vi "DecodePacket.vi"(0 "object in":refnum<class "Referee.lvclass">, 2 "element":u8[](array[numeric]), 5 "error in (no error)":errorcluster) -> (14 "object out":refnum<class "Referee.lvclass">, 16 "Packet out":T1, 19 "error out":errorcluster)   [LabVIEW 2023, in "Referee.lvclass"]
uses:
  Referee.lvclass
  Packet.ctl
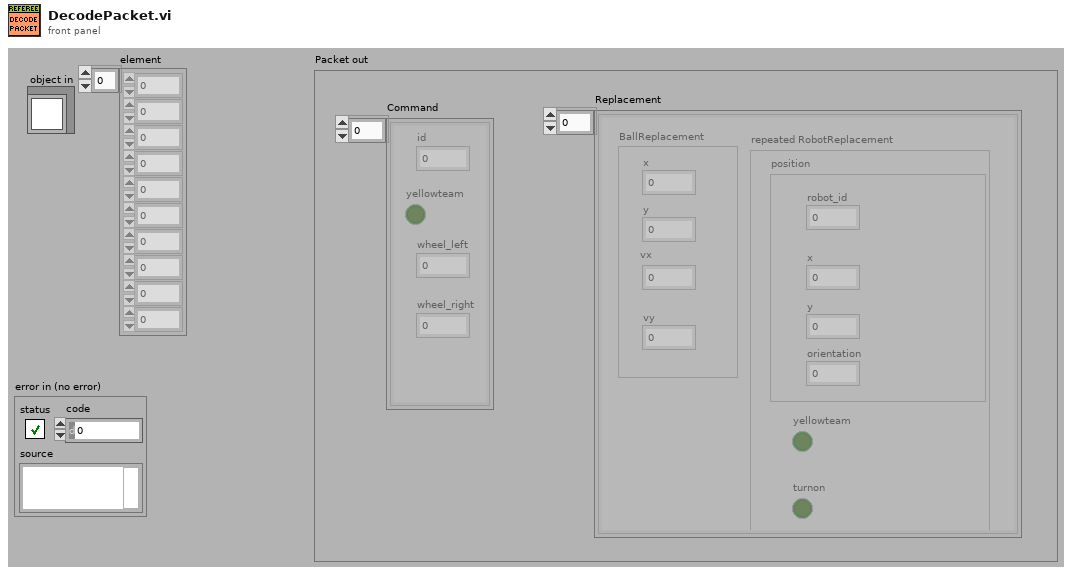
[diagram p1: front panel]
types:
  T1 = typedef "Referee.lvclass/Packet.ctl" = cluster{"Command":cluster{"id":dbl, "yellowteam":bool, "wheel_left":dbl, "wheel_right":dbl}[], "Replacement":cluster{"BallReplacement":cluster{"x":dbl, "y":dbl, "vx":dbl, "vy":dbl}, "repeated RobotReplacement":cluster{"position":cluster{"robot_id":dbl, "x":dbl, "y":dbl, "orientation":dbl}, "yellowteam":bool, "turnon":bool}}[]}
  T2 = cluster{"id":dbl, "yellowteam":bool, "wheel_left":dbl, "wheel_right":dbl}[]
  T3 = cluster{"BallReplacement":cluster{"x":dbl, "y":dbl, "vx":dbl, "vy":dbl}, "repeated RobotReplacement":cluster{"position":cluster{"robot_id":dbl, "x":dbl, "y":dbl, "orientation":dbl}, "yellowteam":bool, "turnon":bool}}[]
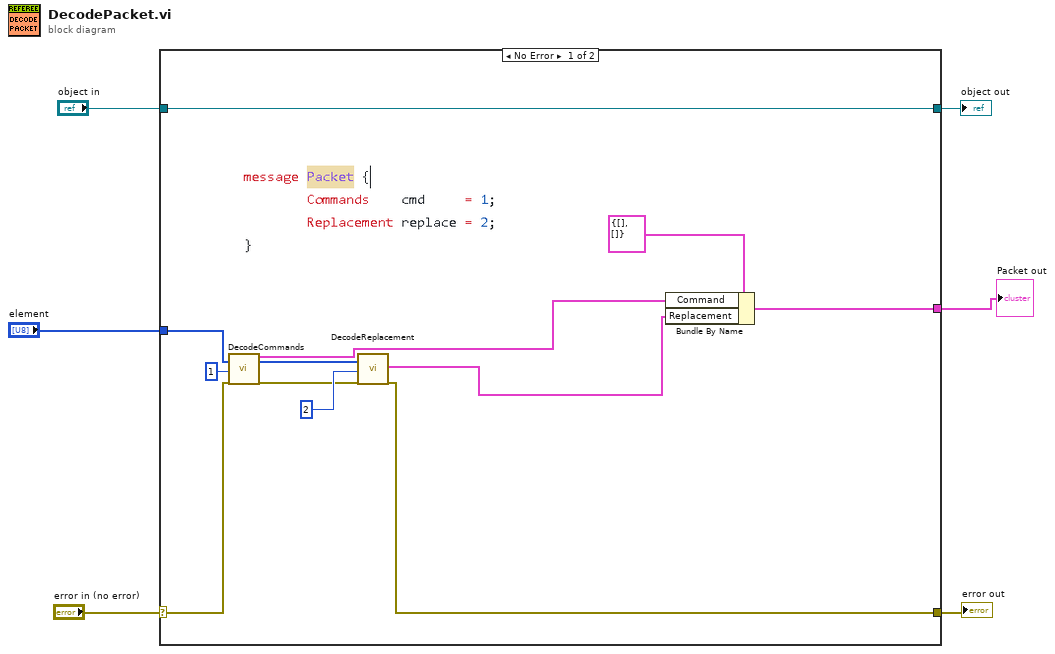
[diagram p0: block diagram]
diagram:
  n1 = case shown="No Error" "error in (no error)" {
    selector: "error in (no error)" -> [w13 w20]
    tunnel: [w12 w20] -> w5
    tunnel: [w18 w19] -> w3
    tunnel: "object in" -> [w18 w19]
    tunnel: "element" -> [w17 _]
    tunnel: [w10 _] -> w1
    frame No Error {
      n2 = call "DecodeCommands.vi"("element"=w17, "Key"=1, "error in (no error)"=w13) -> ("Commands"=w8:T2, "element 2"=w11:u8[], "error out"=w14:errorcluster)  [unwired: 14 in]
      n3 = call "DecodeReplacement.vi"("element"=w11, "Key"=2, "error in (no error)"=w14) -> ("Replacement"=w7:T3, "error out"=w12:errorcluster)  [unwired: 14 in, 1 out]
      n4 = Bundle By Name(cluster=T1 {"Command"=[], "Replacement"=[]} ("Packet out 2"), "Command"=w8, "Replacement"=w7) -> (w10:T1)
    }
    frame Error {
    }
  }
  "error out" <- w5
  "object out" <- w3
  "Packet out" <- w1
